vi "Sig2MS getIonisationSignal.vi"(8 "error in (no error)":errorcluster, 9 "signal in":waveform(sgl), 11 "Sig2MS in":refnum<class "Sig2MS.lvclass">) -> (0 "error out":errorcluster, 3 "Sig2MS out":refnum<class "Sig2MS.lvclass">)   [LabVIEW 2018, in "Sig2MS.lvclass"]
uses:
  Sig2MS.lvclass
  Sig2MS.lvclass/Sig2MS.ctl
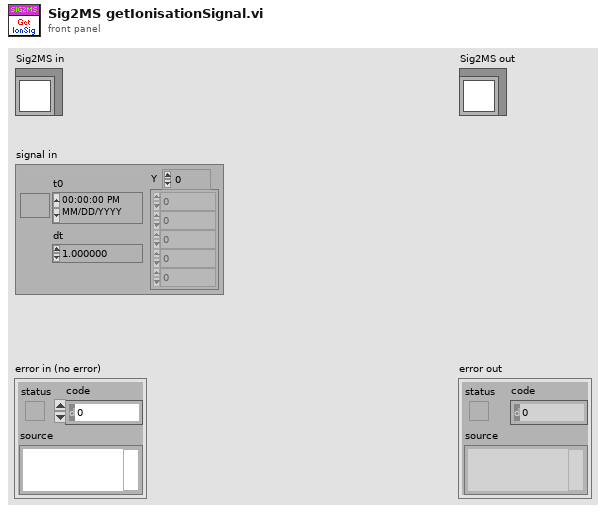
[diagram p1: front panel]
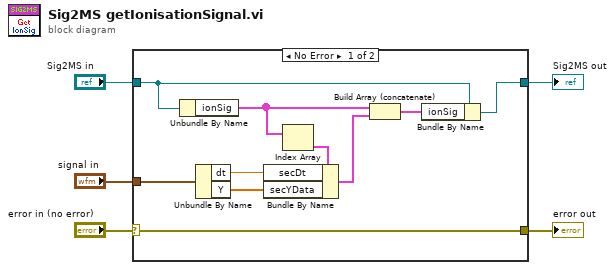
[diagram p0: block diagram]
diagram:
  n1 = case shown="No Error" "error in (no error)" {
    selector: "error in (no error)" -> [w15 w17]
    tunnel: [w15 w17] -> w1
    tunnel: [w14 w16] -> w5
    tunnel: "Sig2MS in" -> [w13 w16]
    tunnel: "signal in" -> [w9 _]
    frame No Error {
      n2 = Unbundle By Name(w13) -> ("ionSig"=w11:cluster{"secDt":dbl, "secYData":sgl[]}[])
      n3 = Unbundle By Name(w9) -> ("dt"=w8:dbl, "Y"=w7:sgl[])
      n4 = Index Array(array=w11) -> (element=w10:cluster{"secDt":dbl, "secYData":sgl[]})  [unwired: 1 in]
      n5 = Bundle By Name(cluster=w10, "secDt"=w8, "secYData"=w7) -> (w6:cluster{"secDt":dbl, "secYData":sgl[]})
      n6 = Build Array (concatenate)(w11, w6) -> (w12:cluster{"secDt":dbl, "secYData":sgl[]}[])
      n7 = Bundle By Name(cluster=w13, "ionSig"=w12) -> (w14:refnum<class "Sig2MS.lvclass">)
    }
    frame Error {
    }
  }
  "error out" <- w1
  "Sig2MS out" <- w5
